vi "main_load_environtment.vi"(6 "Starttime":refnum<vi>, 7 "Env. Dir":refnum<vi>, 8 "Env. Ready?":refnum<vi>, 9 "Env. Tree":refnum<vi>, 10 "Load Env":refnum<vi>, 11 "Running?":refnum<vi>) -> ()   [LabVIEW 2019]
uses:
  <vilib>/Utility/sysdir.llb/System Directory Type.ctl
  lib/libSimulationControl/libSimulationControl.lvlib
panel:
  # "*******************************************************************\nBiogas Plant Control\n\nAuthor: Paul Zügel\nGCSC-Frankfurt am Main 2020\n\n*******************************************************************"
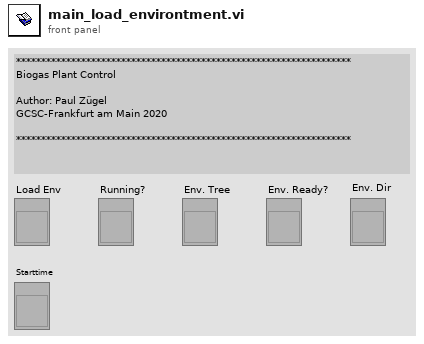
[diagram p1: front panel]
types:
  T1 = enum8{"Enabled", "Disabled", "Disabled and Grayed Out"}
  T2 = cluster{"Left Cell String":string, "Child Text":string[], "Child Tag":string, "Item Indent":i32, "Child Only?":bool, "Glyph Index":i32}
  T3 = typedef "System Directory Type.ctl" = i32
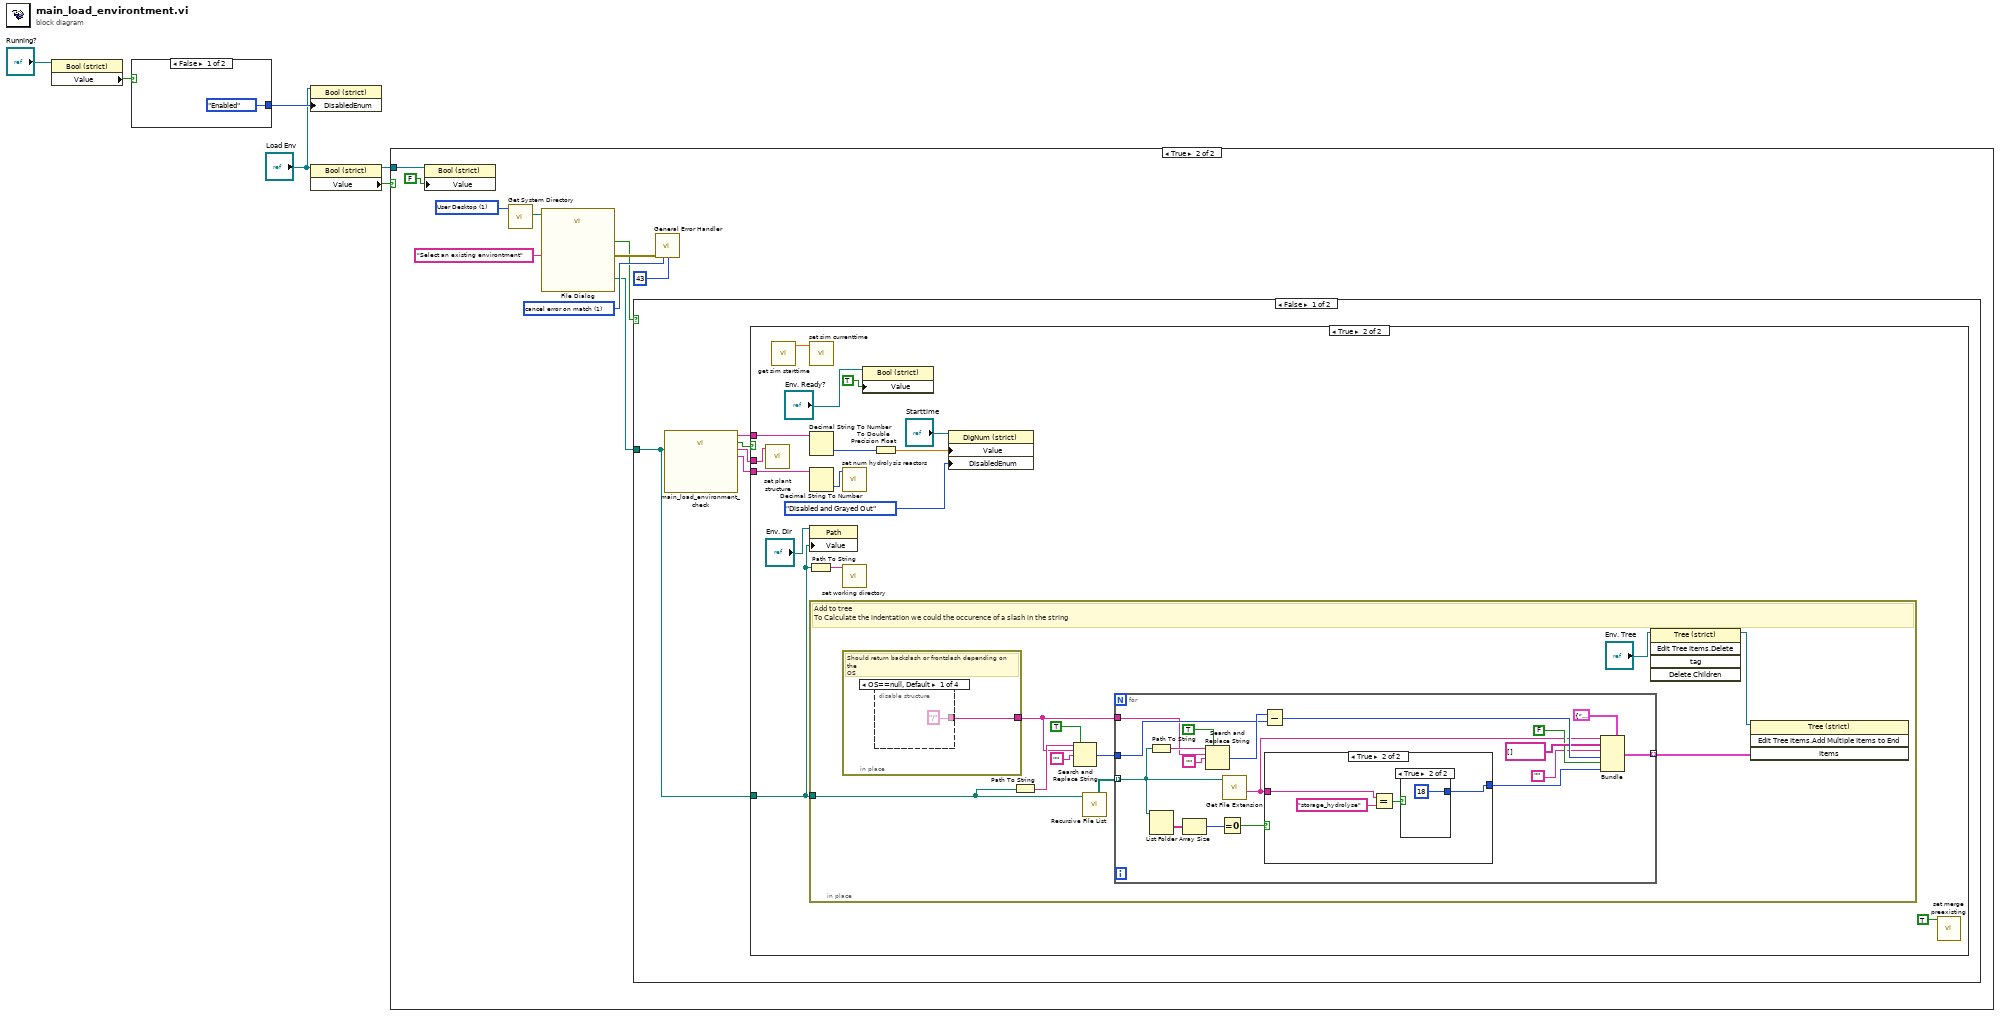
[diagram p0: block diagram]
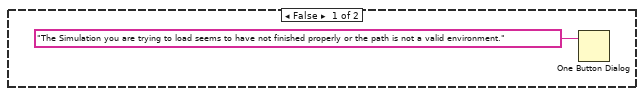
[diagram p3: hidden frame]
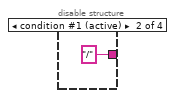
[diagram p4: hidden frame]
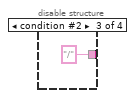
[diagram p5: hidden frame]
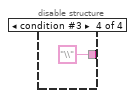
[diagram p6: hidden frame]
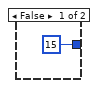
[diagram p7: hidden frame]
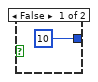
[diagram p8: hidden frame]
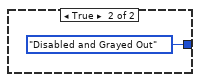
[diagram p10: hidden frame]
diagram:
  n1 = property class="Bool (strict)"(reference="Running?") -> ("Value"=w5:bool)  [unwired: 1 in, 2 out]
  n2 = case shown="False" w5 {
    tunnel: [T1."Enabled" ("Disabled") T1."Disabled and Grayed Out" ("Disabled")] -> w4
    frame False {
    }
    frame True {
    }
  }
  n3 = property class="Bool (strict)"(reference="Load Env", "DisabledEnum"=w4) -> ()  [unwired: 1 in, 2 out]
  n4 = property class="Bool (strict)"(reference="Load Env") -> (reference out=w1:refnum<vi>, "Value"=w2:bool)  [unwired: 1 in, 1 out]
  n5 = case shown="True" w2 {
    tunnel: w1 -> [_ w18]
    frame False {
    }
    frame True {
      w14 = T3 1 items=["User Home"=0, "User Desktop"=1, "User Documents"=2, "User Application Data"=3, "User Preferences"=4, "User Temporary"=5, "Public Documents"=6, "Public Application Data"=7, "Public Preferences"=8, "Public Cache"=13, "System Core Libraries"=9, "System Installed Libraries"=10, "Application Files"=11, "Boot Volume Root"=12] ("system directory type")
      w13 = 1 items=["no exception", "cancel error on match", "set error on match"] ("[exception action] (none:0)")
      n6 = property class="Bool (strict)"(reference=w18, "Value"=FALSE) -> ()  [unwired: 1 in, 2 out]
      n7 = call <vilib>:"Get System Directory.vi"("system directory type"=w14) -> ("system directory"=w16:path)  [unwired: 10 in]
      n8 = call "File Dialog"("start path"=w16, "prompt"="Select an existing environtment") -> ("selected path"=w9:path, "cancelled"=w10:bool, "error out"=w15:errorcluster)  [unwired: 10 in, 1 out]
      n9 = case shown="False" w10 {
        tunnel: w9 -> [w23 _]
        frame False {
          n10 = call "main_load_environment_check.vi"("New working Dir"=w23) -> ("Num_Hydro"=w19:string, "Structure"=w20:string, "Valid?"=w22:bool, "Endtime"=w21:string)  [unwired: 7 in]
          n11 = case shown="True" w22 {
            tunnel: w23 -> [_ w34]
            tunnel: w21 -> [_ w31]
            tunnel: w20 -> [_ w28]
            tunnel: w19 -> [_ w27]
            frame False {
              n12 = One Button Dialog(message="The Simulation you are trying to load seems to have not finished properly or the path is not a valid environment.") -> ()  [unwired: 1 in, 1 out]
            }
            frame True {
              n13 = call "set plant structure.vi"("structure"=w28) -> ()  [unwired: 10 in, 1 out]
              n14 = call "get sim starttime.vi"() -> ("sim_starttime"=w25:dbl)  [unwired: 10 in, 1 out]
              n15 = Path To String(path=w34) -> (string=w39:string)
              n16 = call "set sim currenttime.vi"("time"=w25) -> ()  [unwired: 10 in, 1 out]
              n17 = Decimal String To Number(string=w31) -> (number=w29:i32)  [unwired: 2 in, 1 out]
              n18 = Decimal String To Number(string=w27) -> (number=w26:i32)  [unwired: 2 in, 1 out]
              n19 = property class="Path"(reference="Env. Dir", "Value"=w34) -> ()  [unwired: 1 in, 2 out]
              n20 = in-place {
                in-place-border: w34 -> [w44]
                # "Add to tree\nTo Calculate the indentation we could the occurence of a slash in the string"
                n21 = in-place {
                  in-place-border: [w50] -> w40
                  # "Should return backslash or frontslash depending on the\nOS"
                  n22 = disable-structure shown="OS==null, Default" {
                    disable-tunnel: ["/" ("name or relative path") "/" ("name or relative path") "/" ("name or relative path") "\\" ("name or relative path")] -> w50
                    frame condition #0 {
                    }
                    frame condition #1 (active) {
                    }
                    frame condition #2 {
                    }
                    frame condition #3 {
                    }
                  }
                }
                n23 = Path To String(path=w44) -> (string=w48:string)
                n24 = Search and Replace String(replace all?=TRUE ("replace all? (F)"), input string=w48, search string=w40, replace string="") -> (number of replacements=w45:i32)  [unwired: 4 in, 3 out]
                n25 = call <vilib>:"Recursive File List.vi"("Folder Path"=w44) -> ("All Folders"=w49:path[])  [unwired: 6 in, 4 out]
                n26 = for {
                  tunnel: w49 -> [w58] mode=indexing
                  tunnel: w45 -> [w68]
                  tunnel: [w67] -> w41 mode=indexing
                  tunnel: w40 -> [w55]
                  n27 = Path To String(path=w58) -> (string=w72:string)
                  n28 = List Folder(path=w58) -> (folder names=w57:string[])  [unwired: 3 in, 3 out]
                  n29 = Array Size(array=w57) -> (size(s)=w61:i32)
                  n30 = Search and Replace String(replace all?=TRUE ("replace all? (F)"), input string=w72, search string=w55, replace string="") -> (number of replacements=w69:i32)  [unwired: 4 in, 3 out]
                  n31 = Equal To 0?(x=w61) -> (x = 0?=w60:bool)
                  n32 = call <vilib>:"Get File Extension.vi"("file"=w58) -> ("filename without extension"=w56:string)  [unwired: 6 in, 4 out]
                  n33 = Subtract(x=w69, y=w68) -> (x-y=w66:i32)
                  n34 = case shown="True" w60 {
                    tunnel: [15 ("Glyph Index") w74] -> w59
                    tunnel: w56 -> [_ w77]
                    frame False {
                    }
                    frame True {
                      n35 = Equal?(x=w77, y="storage_hydrolyse") -> (x = y?=w75:bool)
                      n36 = case shown="True" w75 {
                        tunnel: [10 ("Glyph Index") 18 ("Glyph Index")] -> w74
                        frame False {
                        }
                        frame True {
                        }
                      }
                    }
                  }
                  n37 = Bundle(cluster=T2 {"Left Cell String"="", "Child Text"=[], "Child Tag"="", "Item Indent"=0, "Child Only?"=FALSE, "Glyph Index"=0} ("Item"), "Left Cell String"=w56, "Child Text"=string[] [], "Child Tag"="", "Item Indent"=w66, "Child Only?"=FALSE, "Glyph Index"=w59) -> (w67:T2)
                }
                n38 = invoke class="Tree (strict)" method="Edit Tree Items.Delete"(reference="Env. Tree") -> (reference out=w42:refnum<vi>)  [unwired: 4 in, 4 out]
                n39 = invoke class="Tree (strict)" method="Edit Tree Items.Add Multiple Items to End"(reference=w42, "Items"=w41) -> ()  [unwired: 2 in, 4 out]
              }
              n40 = call "set num hydrolysis reactors.vi"("num"=w26) -> ()  [unwired: 10 in, 1 out]
              n41 = call "set working directory.vi"("dir"=w39) -> ()  [unwired: 10 in, 1 out]
              n42 = property class="Bool (strict)"(reference="Env. Ready?", "Value"=TRUE) -> ()  [unwired: 1 in, 2 out]
              n43 = To Double Precision Float(number=w29) -> (double precision float=w30:dbl)
              n44 = property class="DigNum (strict)"(reference="Starttime", "Value"=w30, "DisabledEnum"=T1."Disabled and Grayed Out" ("Disabled")) -> ()  [unwired: 1 in, 2 out]
              n45 = call "set merge preexisting.vi"("merge"=TRUE) -> ()  [unwired: 10 in, 1 out]
            }
          }
        }
        frame True {
        }
      }
      n46 = call <vilib>:"General Error Handler.vi"("error in (no error)"=w15, "[exception action] (none:0)"=w13, "[exception code]"=43) -> ()  [unwired: 8 in, 5 out]
    }
  }
